vi "User_Modify.vi"(10 "User_Name":string caption="用  户  名") -> ()   [LabVIEW 2020]
uses:
  <vilib>/Utility/cursorutil.llb/Set Cursor (Icon Pict).vi
panel:
  in  "Delete":bool
  in  "User_Right":u16(ring) caption="权        限" items=["操作员"=2]
  in  "Confirm Password":string caption="确认密码"
  in  "New Password":string caption="新  密  码"
  in  "Ok":bool
  # "修改用户"
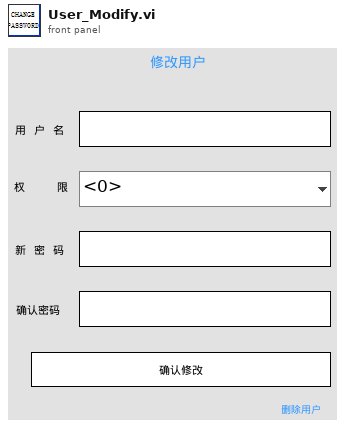
[diagram p1: front panel]
types:
  T1 = typedef "User_Info.ctl" = cluster{"Name":string, "Password":string, "User_Right":u16, "Debuger?":bool, "Manager?":bool, "User_Remember_Name":bool, "User_Remember_PW":bool, "User_Right_String":string, "Null?":bool, "Language":string}
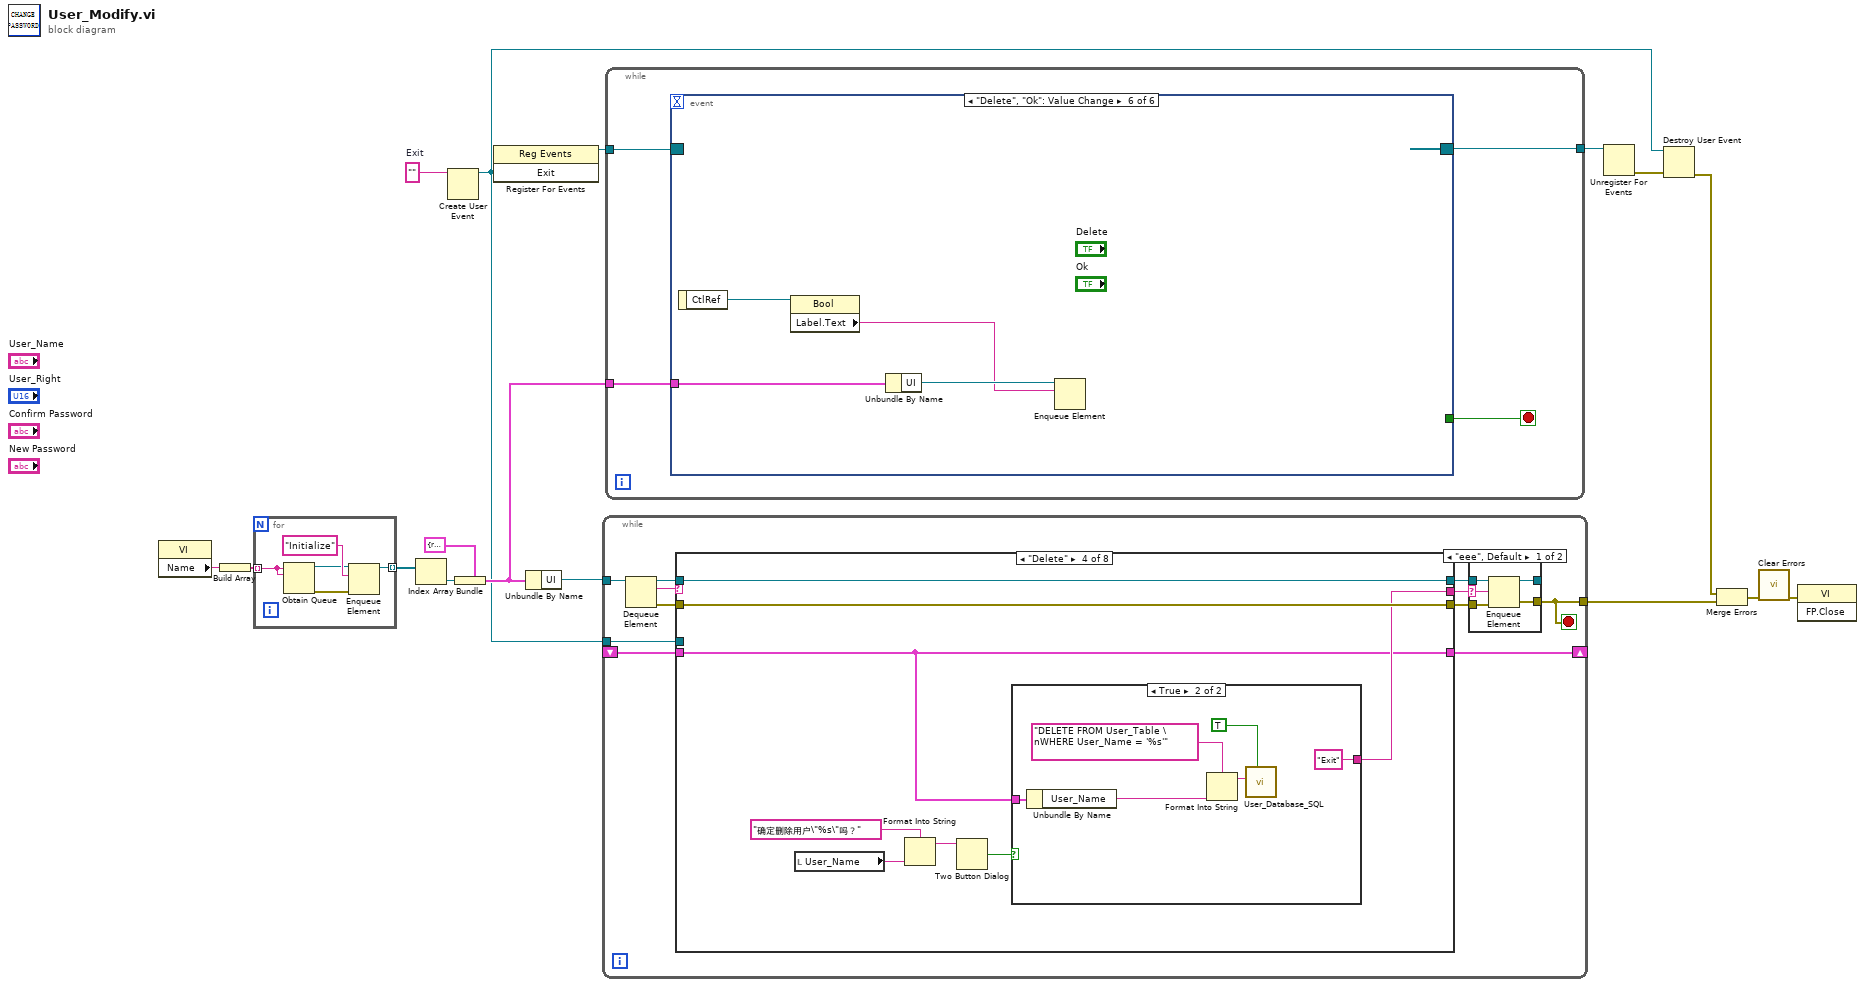
[diagram p0: block diagram]
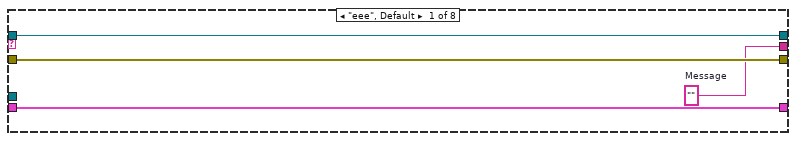
[diagram p3: hidden frame]
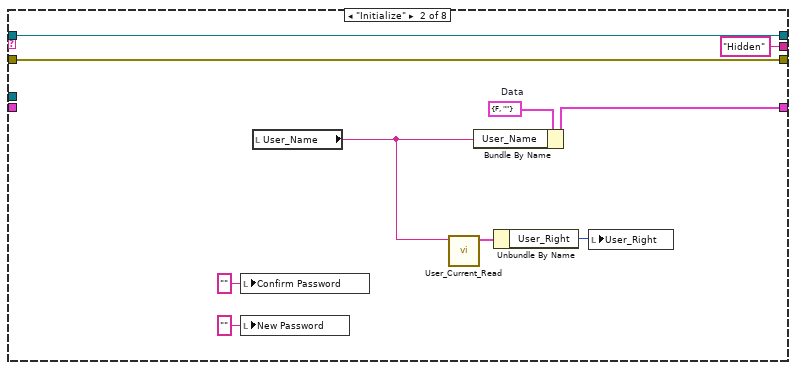
[diagram p4: hidden frame]
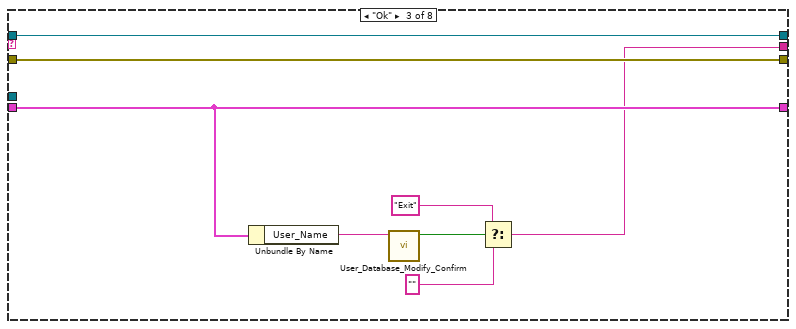
[diagram p5: hidden frame]
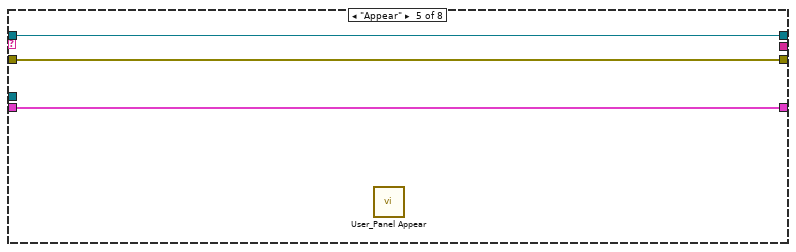
[diagram p7: hidden frame]
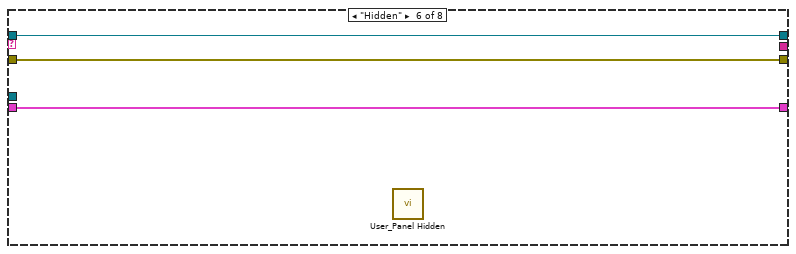
[diagram p8: hidden frame]
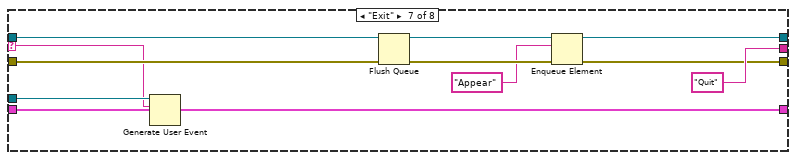
[diagram p9: hidden frame]
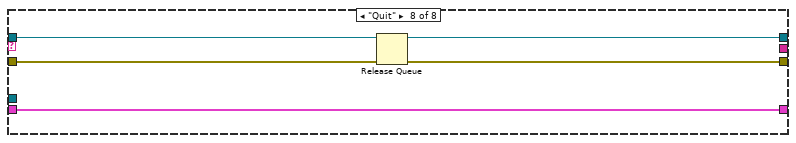
[diagram p10: hidden frame]
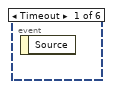
[diagram p11: hidden frame]
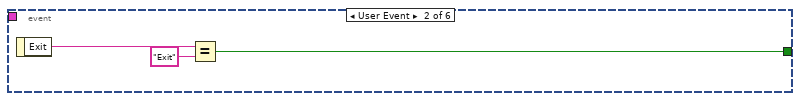
[diagram p12: hidden frame]
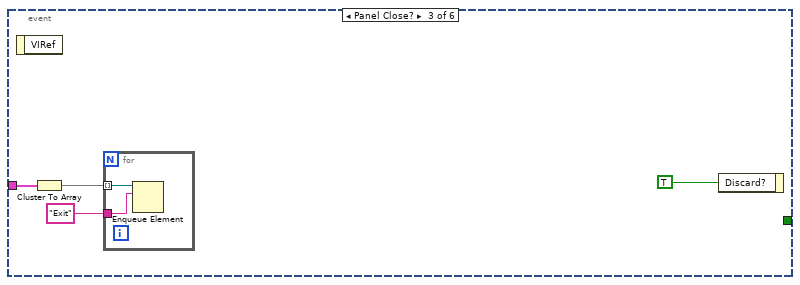
[diagram p13: hidden frame]
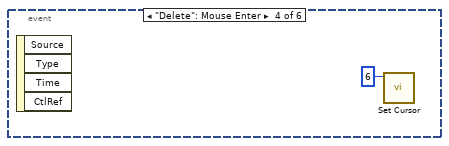
[diagram p14: hidden frame]
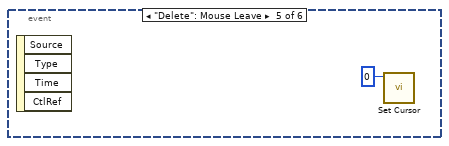
[diagram p15: hidden frame]
diagram:
  w2 = ""  # Exit
  n1 = property class="VI"() -> ("Name"=w12:string)  [unwired: 2 in, 2 out]
  n2 = Build Array(w12) -> (w13:string[])
  n3 = for {
    tunnel: w13 -> [w17] mode=indexing
    tunnel: [w18] -> w7 mode=indexing
    n4 = Obtain Queue(name (unnamed)=w17, element data type=w17) -> (queue out=w20:refnum<queue>, error out=w19:errorcluster)  [unwired: 3 in, 1 out]
    n5 = Enqueue Element(queue=w20, element="Initialize" ("元素"), error in (no error)=w19) -> (queue out=w18:refnum<queue>)  [unwired: 1 in, 2 out]
  }
  n6 = Index Array(array=w7) -> (element=w10:refnum<queue>)  [unwired: 1 in]
  n7 = Create User Event(user event datatype=w2) -> (user event=w6:refnum<user-event>)  [unwired: 1 in, 1 out]
  n8 = Bundle(cluster=cluster{"UI":refnum<queue>} {"UI"=refnum}, "UI"=w10) -> (w11:cluster{"UI":refnum<queue>})
  n9 = register-events(w6) -> (reference out=w3:refnum<event-registration>)  [unwired: 2 in, 1 out]
  n10 = Unbundle By Name(w11) -> ("UI"=w8:refnum<queue>)
  n11 = while {
    tunnel: w8 -> [w32]
    tunnel: [w22] -> w15
    shift-right: [w26] -> _
    shift-left: _ -> [w25]
    tunnel: w6 -> [w24]
    stop <- w22 stop-if-true
    n12 = Dequeue Element(queue=w32) -> (queue out=w31:refnum<queue>, element=w23:string, error out=w28:errorcluster)  [unwired: 2 in, 1 out]
    n13 = case shown="\"Delete\"" w23 {
      selector: w23 -> [_ _ _ _ _ _ w87 _]
      tunnel: w31 -> [w43 w53 w61 w69 w78 w81 w90 w96]
      tunnel: [w43 w53 w61 w69 w78 w81 w83 w96] -> w30
      tunnel: [w42 w52 w60 w68 w77 w80 w84 w93] -> w29
      tunnel: w28 -> [w42 w52 w60 w68 w77 w80 w89 w95]
      tunnel: [w41 "Hidden" ("Message") w54 w63 _ _ "Quit" ("Message") _] -> w27
      tunnel: [w40 w49 w59 w62 w76 w79 w92 w94] -> w26
      tunnel: w25 -> [w40 _ w59 w62 w76 w79 w92 w94]
      tunnel: w24 -> [_ _ _ _ _ _ w88 _]
      frame "eee", Default {
        w41 = ""  # Message
      }
      frame "Initialize" {
        w51 = cluster{"Data":bool, "User_Name":string} {"Data"=FALSE, "User_Name"=""}  # Data
        n14 = local write "Confirm Password"("" ("Confirm Password")) -> ()
        n15 = local write "New Password"("" ("New Password")) -> ()
        n16 = local read "User_Name"() -> (w48:string)
        n17 = call "User_Current_Read.vi"("Name"=w48) -> ("User_Info"=w47:T1)  [unwired: 9 in, 1 out]
        n18 = Bundle By Name(cluster=w51, "User_Name"=w48) -> (w49:cluster{"Data":bool, "User_Name":string})
        n19 = Unbundle By Name(w47) -> ("User_Right"=w46:u16)
        n20 = local write "User_Right"(w46) -> ()
      }
      frame "Ok" {
        n21 = Unbundle By Name(w59) -> ("User_Name"=w58:string)
        n22 = call "User_Database_Modify_Confirm.vi"("Last_User_Name"=w58) -> ("OK"=w57:bool)  [unwired: 9 in, 1 out]
        n23 = Select(t="Exit", s=w57, f="") -> (s? t:f=w54:string)
      }
      frame "Delete" {
        n24 = local read "User_Name"() -> (w66:string)
        n25 = Format Into String(format string="确定删除用户\"%s\"吗？" ("消息"), w66) -> (resulting string=w65:string)  [unwired: 2 in, 1 out]
        n26 = Two Button Dialog(message=w65) -> (T button?=w64:bool)  [unwired: 2 in]
        n27 = case shown="True" w64 {
          tunnel: [_ "Exit"] -> w63
          tunnel: w62 -> [_ w71]
          frame False {
          }
          frame True {
            n28 = Unbundle By Name(w71) -> ("User_Name"=w70:string)
            n29 = Format Into String(format string="DELETE FROM User_Table \nWHERE User_Name = '%s'" ("SQL query"), w70) -> (resulting string=w75:string)  [unwired: 2 in, 1 out]
            n30 = call "User_Database_SQL.vi"("Get Record"=TRUE, "SQL query"=w75) -> ()  [unwired: 7 in, 3 out]
          }
        }
      }
      frame "Appear" {
        n31 = call "User_Panel Appear.vi"() -> ()  [unwired: 11 in, 1 out]
      }
      frame "Hidden" {
        n32 = call "User_Panel Hidden.vi"() -> ()  [unwired: 11 in, 1 out]
      }
      frame "Exit" {
        n33 = Generate User Event(user event=w88, event data cluster=w87) -> ()  [unwired: 2 in, 2 out]
        n34 = Flush Queue(queue=w90, error in (no error)=w89) -> (queue out=w86:refnum<queue>, error out=w85:errorcluster)  [unwired: 1 out]
        n35 = Enqueue Element(queue=w86, element="Appear" ("元素"), error in (no error)=w85) -> (queue out=w83:refnum<queue>, error out=w84:errorcluster)  [unwired: 1 in, 1 out]
      }
      frame "Quit" {
        n36 = Release Queue(queue=w96, error in (no error)=w95) -> (error out=w93:errorcluster)  [unwired: 1 in, 2 out]
      }
    }
    n37 = case shown="\"eee\", Default" w27 {
      selector: w27 -> [w33 _]
      tunnel: w30 -> [w37 w39]
      tunnel: w29 -> [w36 w38]
      tunnel: [w35 w38] -> w22
      tunnel: [w34 w39] -> _
      frame "eee", Default {
        n38 = Enqueue Element(queue=w37, element=w33, error in (no error)=w36) -> (queue out=w34:refnum<queue>, error out=w35:errorcluster)  [unwired: 1 in, 1 out]
      }
      frame "" {
      }
    }
  }
  n39 = while {
    tunnel: w3 -> [w99]
    tunnel: [w98] -> w5
    tunnel: w11 -> [w97]
    stop <- w100 stop-if-true
    n40 = event shown="[5] \"Delete\", \"Ok\": Value Change" {
      selector: w99 -> [_ _ _ _ _ _]
      dyn-events: [_ _ _ _ _ _] -> w98
      timeout: _ -> [_ _ _ _ _ _]
      tunnel: [_ w102 _ _ _ _] -> w100
      tunnel: w97 -> [_ _ w106 _ _ w114]
      event Timeout {
        n41 = event-data() -> ()  [unwired: 1 in, 1 out]
      }
      event User Event {
        n42 = event-data() -> ("Exit"=w103:string)  [unwired: 1 in]
        n43 = Equal?(x=w103, y="Exit") -> (x = y?=w102:bool)
      }
      event Panel Close? {
        n44 = event-data() -> ()  [unwired: 1 in, 1 out]
        n45 = Cluster To Array(cluster=w106) -> (array=w105:refnum<queue>[])
        n46 = for {
          tunnel: w105 -> [w109] mode=indexing
          tunnel: "Exit" ("元素") -> [w108]
          n47 = Enqueue Element(queue=w109, element=w108) -> ()  [unwired: 2 in, 3 out]
        }
        n48 = event-data("Discard?"=TRUE ("放弃？")) -> ()  [unwired: 1 in, 1 out]
      }
      event "Delete": Mouse Enter {
        n49 = event-data() -> ()  [unwired: 1 in, 4 out]
        n50 = call-poly <vilib>:"Set Cursor.vi"("icon"=u16 6) -> ()  [unwired: 9 in, 2 out]
      }
      event "Delete": Mouse Leave {
        n51 = event-data() -> ()  [unwired: 1 in, 4 out]
        n52 = call-poly <vilib>:"Set Cursor.vi"("icon"=u16 0) -> ()  [unwired: 9 in, 2 out]
      }
      event "Delete", "Ok": Value Change {
        n53 = event-data() -> ("CtlRef"=w115:refnum<vi>)  [unwired: 1 in]
        n54 = property class="Bool"(reference=w115) -> ("Label.Text"=w112:string)  [unwired: 1 in, 2 out]
        n55 = Unbundle By Name(w114) -> ("UI"=w113:refnum<queue>)
        n56 = Enqueue Element(queue=w113, element=w112) -> ()  [unwired: 2 in, 3 out]
      }
    }
  }
  n57 = Unregister For Events(event registration refnum=w5) -> (error out=w4:errorcluster)  [unwired: 1 in]
  n58 = Destroy User Event(user event=w6, error in=w4) -> (error out=w14:errorcluster)
  n59 = Merge Errors(w14, w15) -> (w16:errorcluster)
  n60 = call <vilib>:"Clear Errors.vi"("error in (no error)"=w16) -> ("error out"=w1:errorcluster)  [unwired: 5 in, 1 out]
  n61 = invoke class="VI" method="FP.Close"(error in=w1) -> ()  [unwired: 2 in, 3 out]
